vi "Initialize.vi"(8 "error in":errorcluster, 10 "Device":string) -> (0 "error out":errorcluster, 3 "Control Box out":refnum<class "Control Box.lvclass">)   [LabVIEW 2018, in "Control Box.lvlib" / "Control Box.lvclass"]
uses:
  Control Box.lvclass
  Control Box.lvclass/Control Box.ctl
  builds/Configuration.lvlibp/Configuration.lvclass
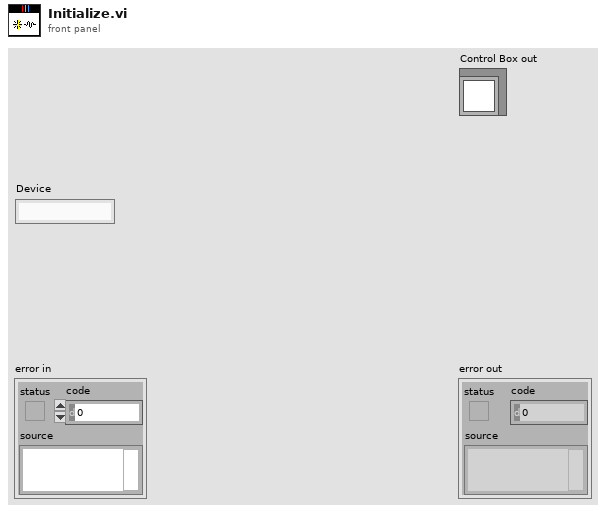
[diagram p1: front panel]
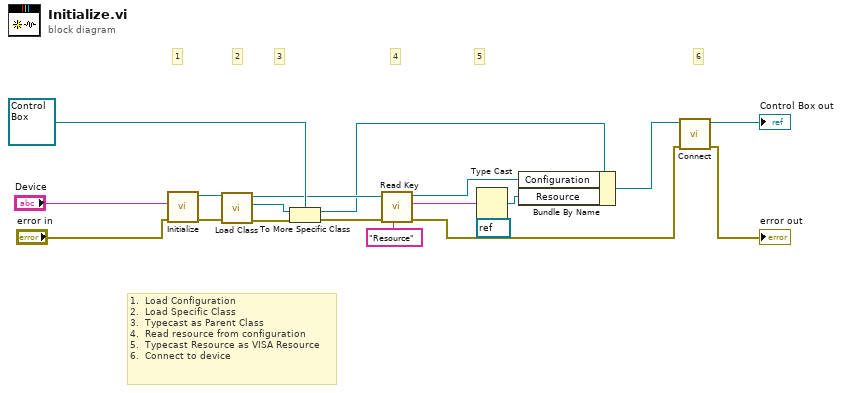
[diagram p0: block diagram]
diagram:
  # "1.  Load Configuration\n2.  Load Specific Class\n3.  Typecast as Parent Class\n4.  Read resource from configuration\n5.  Typecast Resource as VISA Resource\n6.  Connect to device"
  # "6"
  # "5"
  # "4"
  # "3"
  # "2"
  # "1"
  n1 = call "Initialize.vi"("error in"="error in", "Device"="Device") -> ("error out"=w18:errorcluster, "Configuration out"=w19:refnum<class "Configuration.lvclass">)  [unwired: 8 in]
  n2 = call "Load Class.vi"("error in"=w18, "Configuration in"=w19) -> ("error out"=w16:errorcluster, "Class out"=w15:refnum<class>, "Configuration out"=w13:refnum<class "Configuration.lvclass">)  [unwired: 7 in]
  n3 = To More Specific Class(target class=refnum<class "Control Box.lvclass"> refnum ("Control Box in"), reference=w15, error in=w16) -> (specific class reference=w11:refnum<class "Control Box.lvclass">, error out=w12:errorcluster)
  n4 = call "Read Key.vi"("Key:"="Resource", "error in"=w12, "Configuration in"=w13) -> ("error out"=w2:errorcluster, "Value"=w9:string, "Configuration out"=w6:refnum<class "Configuration.lvclass">)  [unwired: 6 in]
  n5 = Type Cast(type=refnum<visa-resource-name> refnum ("Resource"), x=w9) -> (*(type *) &x=w7:refnum<visa-resource-name>)
  n6 = Bundle By Name(cluster=w11, "Configuration"=w6, "Resource"=w7) -> (w4:refnum<class "Control Box.lvclass">)
  n7 = call-dynamic "Connect.vi"("error in"=w2, "Control Box in"=w4) -> ("error out"=→"error out":errorcluster, "Control Box out"=→"Control Box out":refnum<class "Control Box.lvclass">)  [unwired: 8 in]
